vi "load_target.vi"() -> ()   [LabVIEW 2015]
uses:
  subvi/controls.llb/command.ctl
  <vilib>/Platform/TimedLoop/XDataNode/timing_clust.ctl
  <vilib>/Platform/TimedLoop/XDataNode/nitl_modes.ctl
  <vilib>/Platform/TimedLoop/XDataNode/wakeup.ctl
  subvi/controls.llb/RTFIFO operate.ctl
  subvi/Enum data queue_Ctrls.ctl
  <vilib>/addons/control/pid/pid.llb/PID (DBL).vi
  <vilib>/platform/TimedLoop/XDataNode/XDataNode.xnode
  subvi/event data queues.lvlib
  <vilib>/Platform/TimedLoop/XDataNode/XDNodeRunTimeDep.lvlib
  <vilib>/addons/control/pid/NI_PID_pid.lvlib
panel:
  out "T":dbl
  out "data":T1
  out "pat":T2
  out "Sin_MODE_RUN state 2":string
  out "Sin_MODE_RUN state":string
  out "doing":T3(ring)
  out "Boolean array":bool[](array[boolean])
  out "length 2":i32
  out "length":i32
  out "运行":string
  out "state":T3(ring)
  out "exit":bool=TRUE
  in  "variable":T5 {"command" items=["NO_Action", "start", "pause", "resum", "stop", "config"]}
  in  "error in":errorcluster
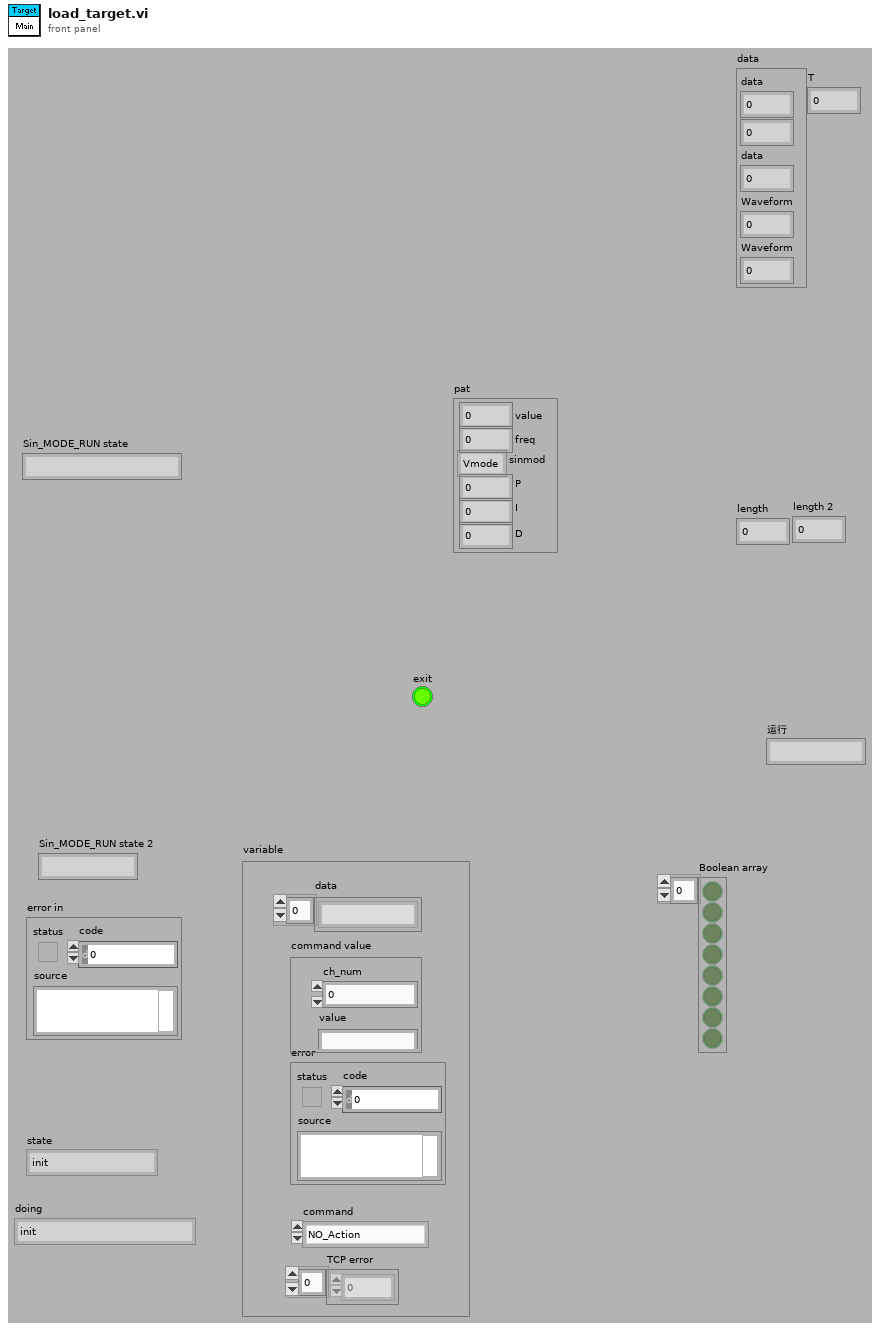
[diagram p1: front panel]
types:
  T1 = cluster{"data":dbl, dbl, "data":u8, "Waveform":dbl, "Waveform":dbl}
  T2 = cluster{"value":dbl, "freq":dbl, "sinmod":enum16{"Vmode", "Tmode", "PIDTmode"}, "P":dbl, "I":dbl, "\nD":dbl}
  T3 = enum16{"init", "wait", "start", "do", "stop", "exit"}
  T4 = typedef "command.ctl" = u16
  T5 = cluster{"error":errorcluster, "TCP error":i32[], "command":T4, "command value":cluster{"ch_num":dbl, "value":string}, "data":string[]}
  T6 = typedef "XDNodeRunTimeDep.lvlib/timing_clust.ctl" = cluster{"Expected End [f-1]":u64, "Actual End [f-1]":u64, "Finished Late? [f-1]":bool, "Expected End [i-1]":u64, "Actual End [i-1]":u64, "Finished Late? [i-1]":bool, "Expected Start [i]":u64, "Actual Start [i]":u64, "Expected Start [f]":u64, "Actual Start [f]":u64, "Source Name":string, "Structure Name":string, "Period":i64, "Deadline":i64, "Offset":i64, "Start":i64, "Priority":i32, "Timeout":i32, "Mode":T7, "Wakeup Reason":T8, "Error":errorcluster, "Source Type":string, "Secondary Source Type":string, "Global End Time":u64, "Global Start Time":u64, "Frame Duration":u64, "Iteration Duration":u64, "Assigned CPU":i32, "I/O Scan Engine Mode":u32}
  T7 = typedef "XDNodeRunTimeDep.lvlib/nitl_modes.ctl" = enum32{"No Change", "Process missed periods, maintain original phase", "Discard missed periods, maintain original phase", "Process missed periods, ignore original phase", "Discard missed periods, ignore original phase"}
  T8 = typedef "XDNodeRunTimeDep.lvlib/wakeup.ctl" = enum32{"Normal", "Aborted", "Asynchronous wakeup", "Timing source error", "Timed loop error", "Timeout"}
  T9 = enum16{"init", "config", "start", "write", "stop"}
  T10 = enum16{"init", "config", "start", "read", "stop"}
  T11 = enum16{"connect", "receive data", "send data", "data transfer", "close"}
  T12 = cluster{"data":dbl, dbl, "data":u8, dbl, "mean":dbl}
  T13 = cluster{"data":dbl, "seconds since 1Jan1904":timestamp}
  T14 = enum16{"connect", "receive data", "send data", "data transfer"}
  T15 = cluster{"value":dbl, "freq":dbl, "sinmod":enum16{"Vmode", "Tmode", "PIDTmode"}, "P":dbl, "I":dbl, "D":dbl}
  T16 = typedef "RTFIFO operate.ctl" = enum16{"Creat", "Write", "Read", "Delete"}
  T17 = typedef "event data queues.lvlib/Enum data queue_Ctrls.ctl" = enum16{"Noop", "Send Pro1", "Send data", "Get Pro1", "Get data", "Flush Pro1", "Flush data", "Destroy Pro1", "Destroy data"}
  T18 = cluster{"proportional gain (Kc)":dbl, "integral time (Ti, min)":dbl, "derivative time (Td, min)":dbl}
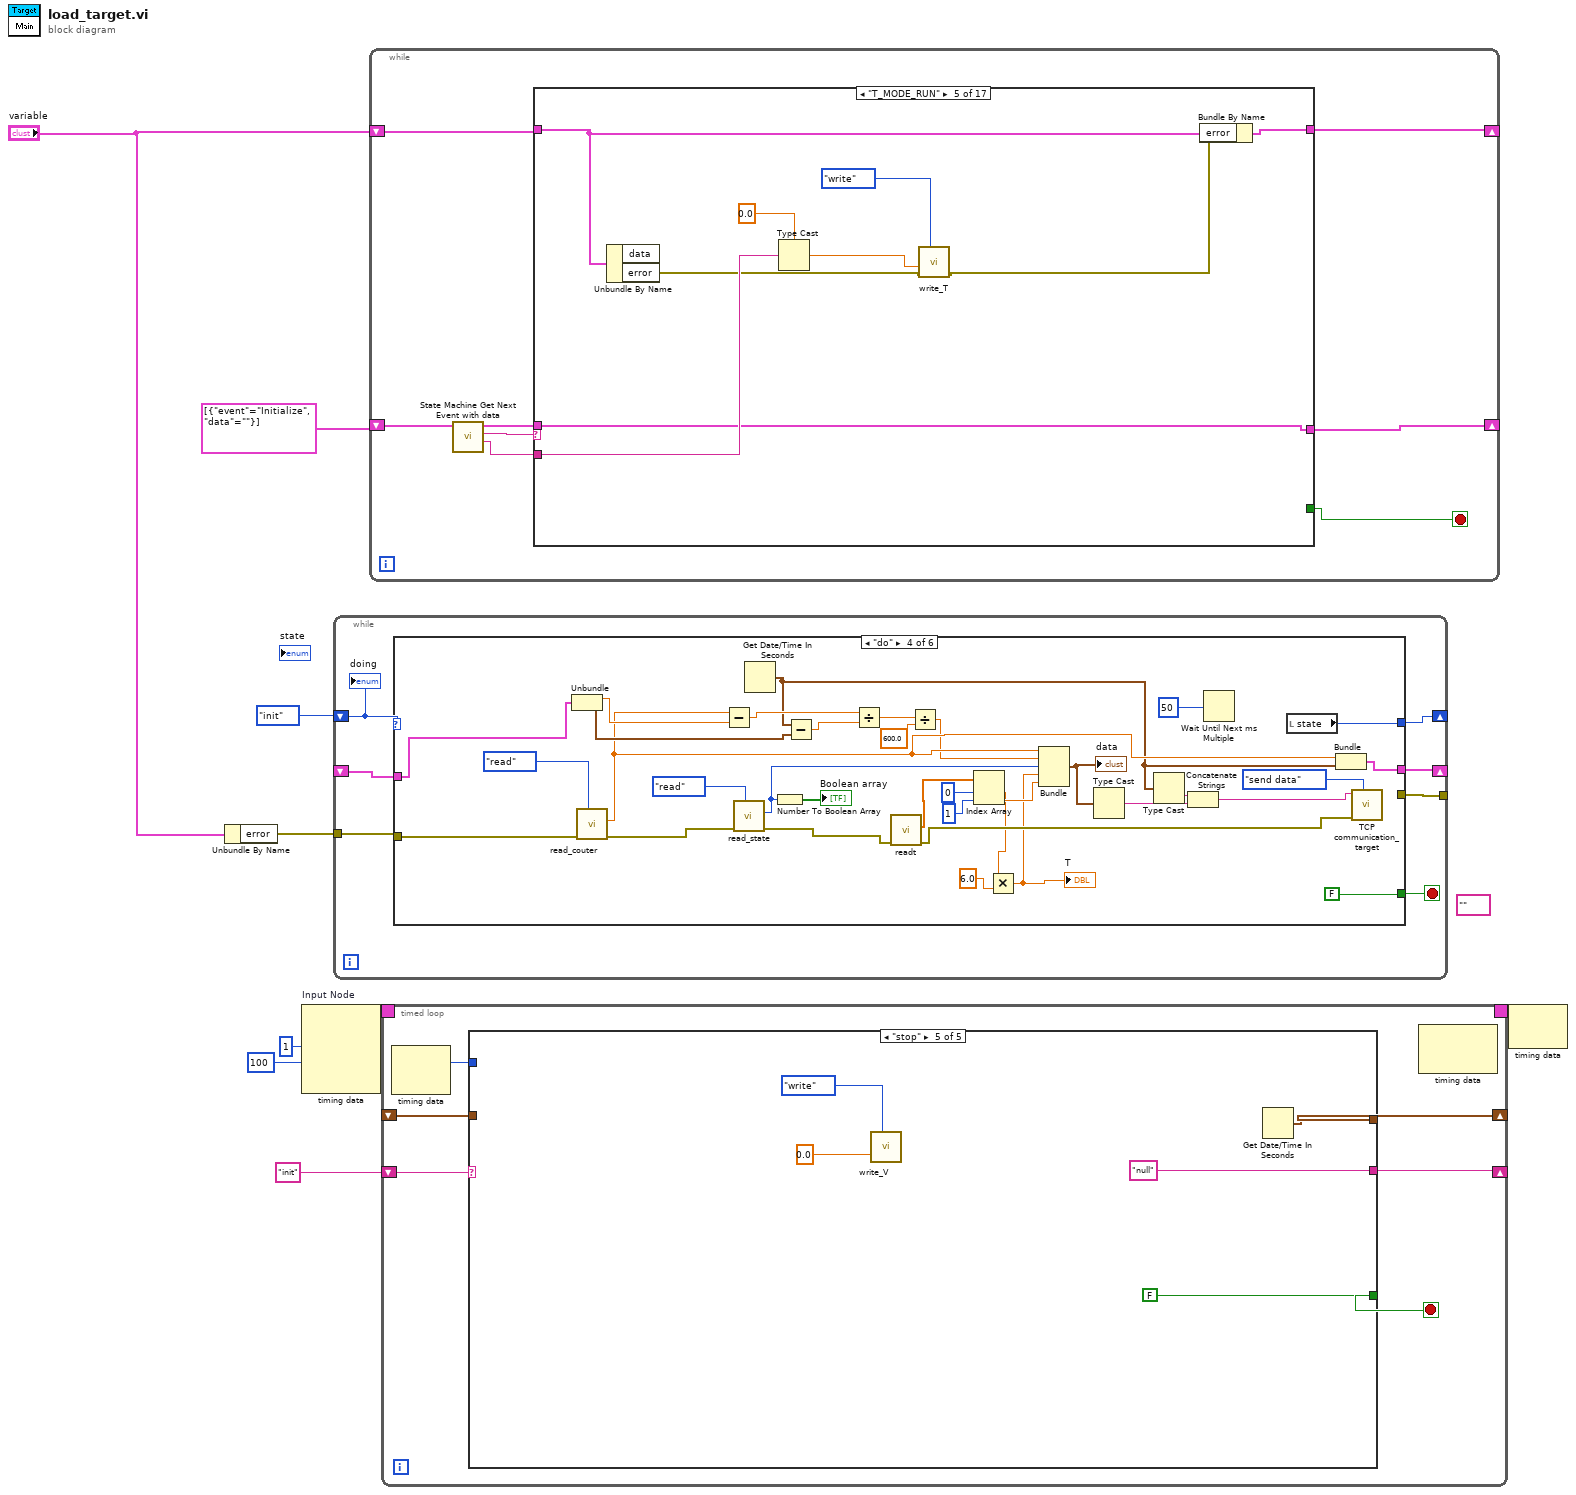
[diagram p0: block diagram]
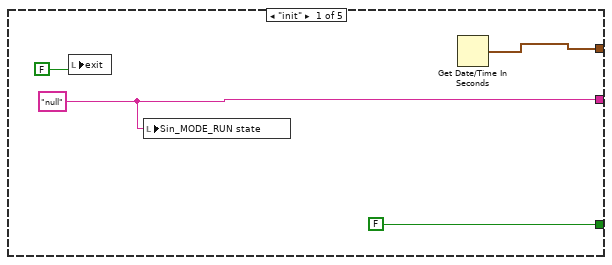
[diagram p2: hidden frame]
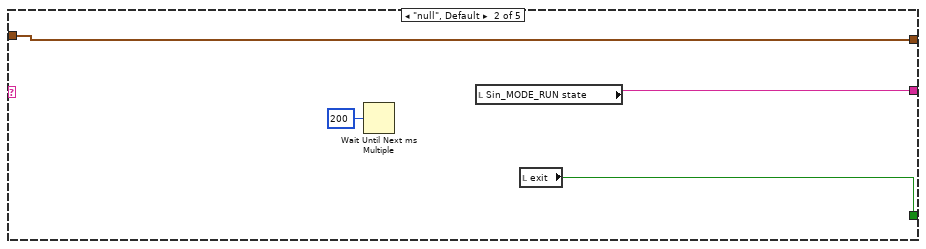
[diagram p3: hidden frame]
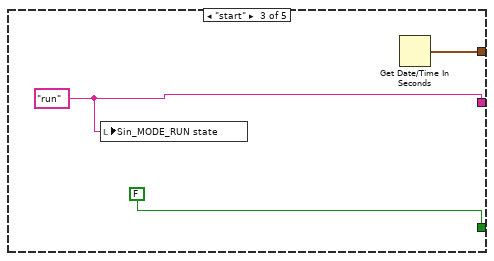
[diagram p4: hidden frame]
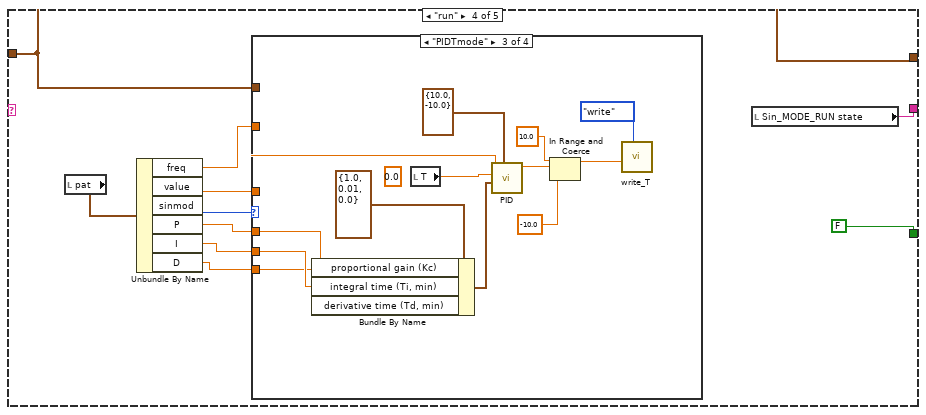
[diagram p5: hidden frame]
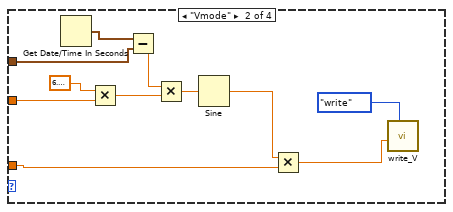
[diagram p7: hidden frame]
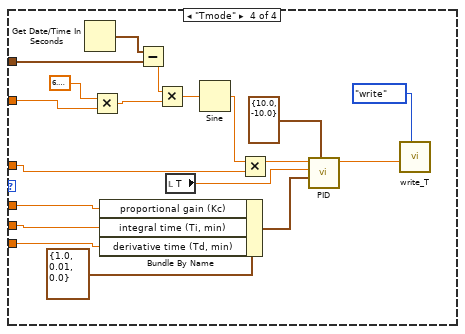
[diagram p8: hidden frame]
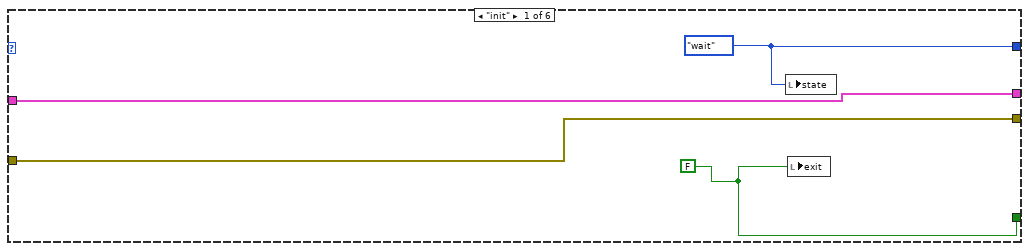
[diagram p9: hidden frame]
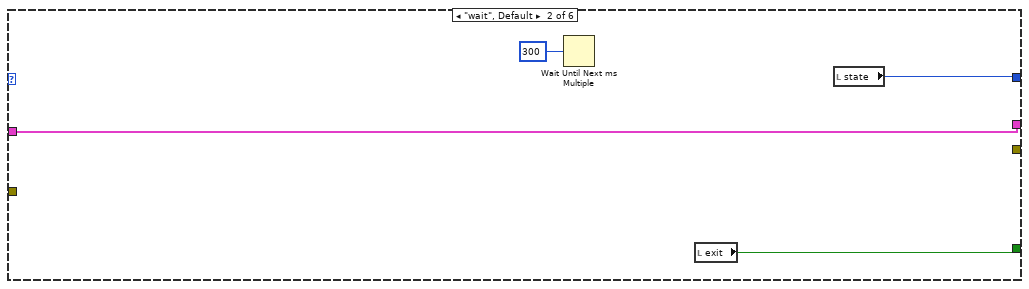
[diagram p10: hidden frame]
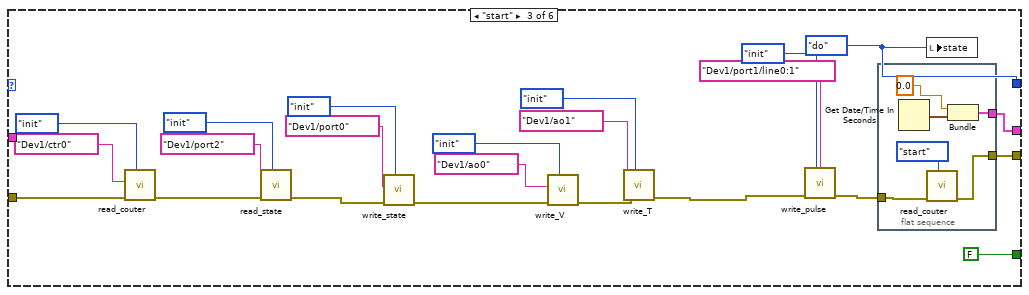
[diagram p11: hidden frame]
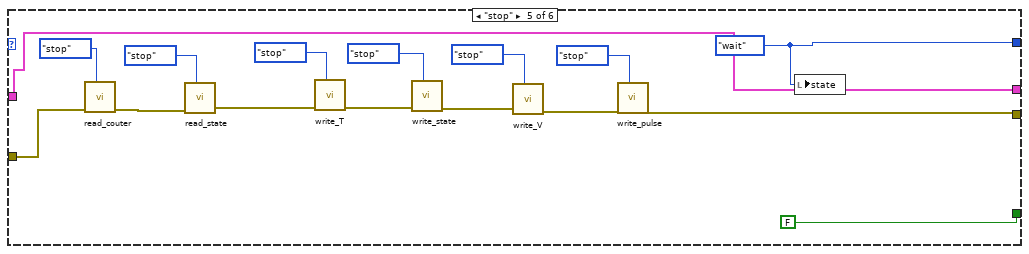
[diagram p12: hidden frame]
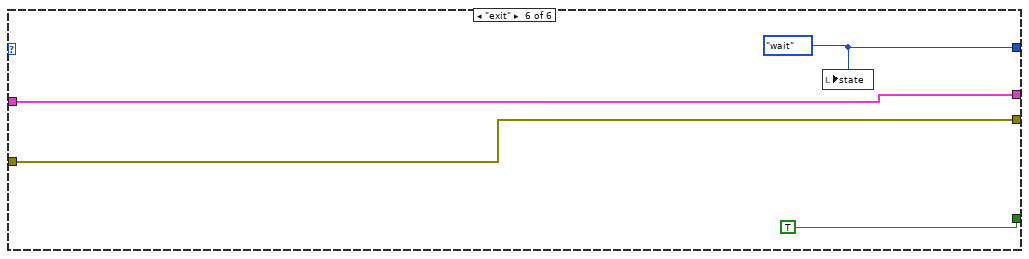
[diagram p13: hidden frame]
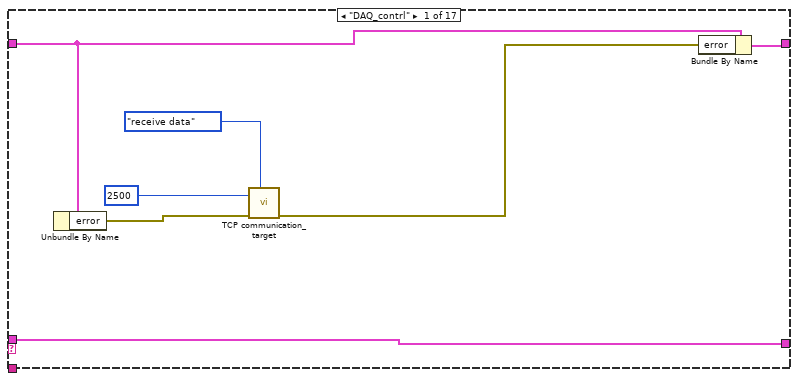
[diagram p14: hidden frame]
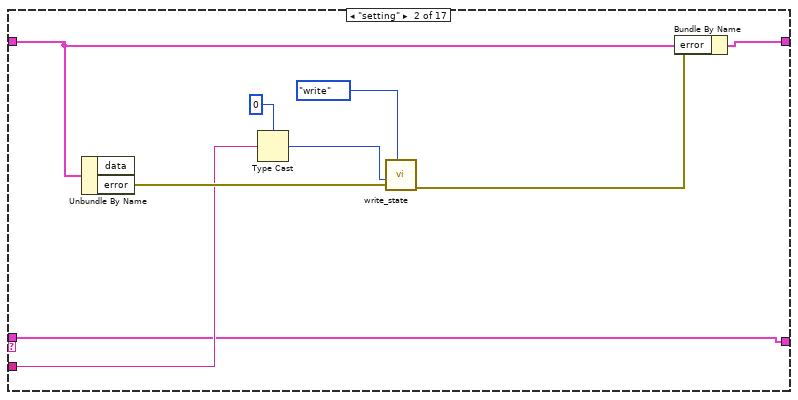
[diagram p15: hidden frame]
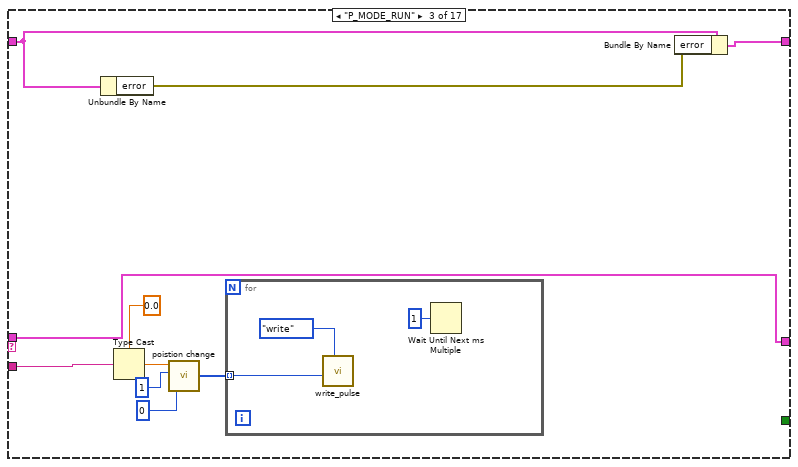
[diagram p16: hidden frame]
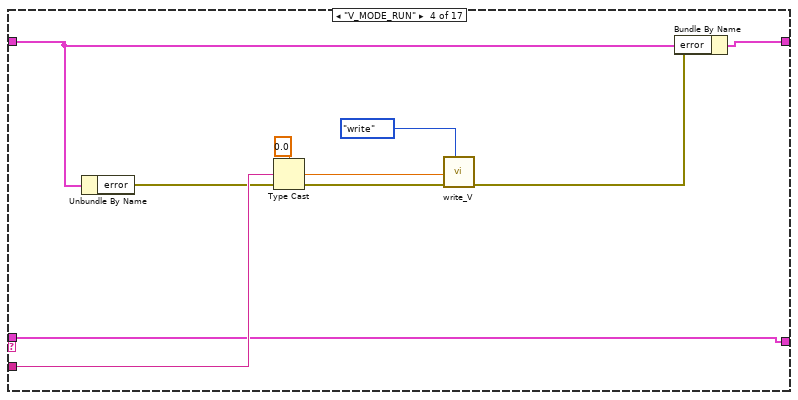
[diagram p17: hidden frame]
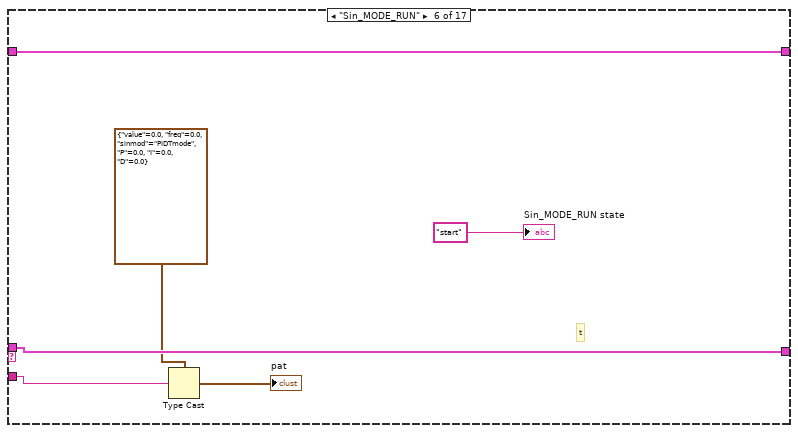
[diagram p18: hidden frame]
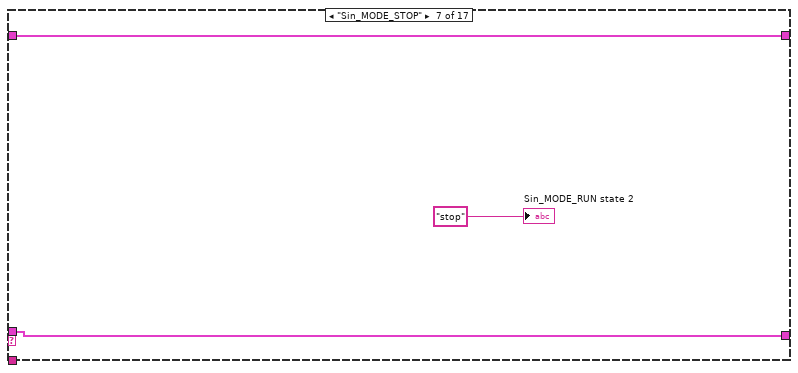
[diagram p19: hidden frame]
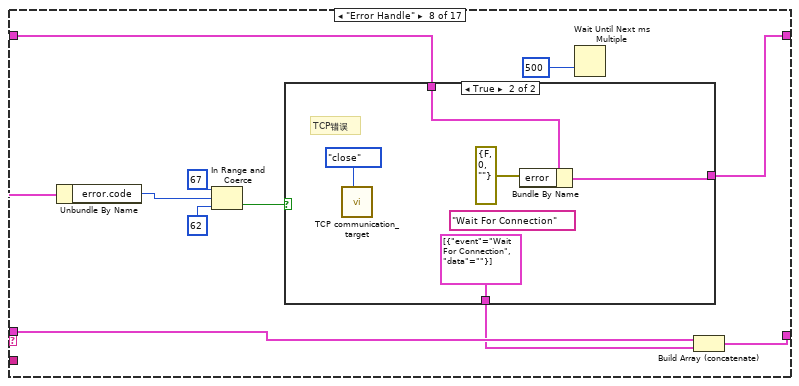
[diagram p20: hidden frame]
diagram:
  (unwired) tag "" ("physical channels")
  n1 = Unbundle By Name("variable") -> ("error"=w8:errorcluster)
  n2 = node-c288 "Input Node"(1 ("Priority"), i64 100 ("Period")) -> (w5:T6)  [unwired: 2 in]
  n3 = while {
    shift-right: [w14] -> _
    shift-left: T3."init" ("Enum") -> [w16]
    tunnel: w8 -> [w13]
    tunnel: [w12] -> _
    shift-right: [w11] -> _
    shift-left: _ -> [w10]
    stop <- w15 stop-if-true
    n4 = case shown="\"do\"" w16 {
      tunnel: [w20 w24 FALSE ("exit") FALSE ("exit") FALSE ("exit") TRUE ("exit")] -> w15
      tunnel: [w19 w23 w46 w86 w102 w106] -> w14
      tunnel: w13 -> [w18 _ w43 w85 w101 w105]
      tunnel: [w18 _ w35 _ w88 w105] -> w12
      tunnel: [w17 w21 w27 w69 w89 w104] -> w11
      tunnel: w10 -> [w17 w21 _ w73 w89 w104]
      frame "init" {
        w19 = T3."wait" ("Enum")
        w20 = FALSE
        n5 = local write "state"(w19) -> ()
        n6 = local write "exit"(w20) -> ()
      }
      frame "wait", Default {
        n7 = Wait Until Next ms Multiple(millisecond multiple=u32 300) -> ()  [unwired: 1 out]
        n8 = local read "exit"() -> (w24:bool)
        n9 = local read "state"() -> (w23:T3)
      }
      frame "start" {
        w46 = T3."do" ("Enum")
        n10 = call "read_couter.vi"("Enum"=T10."init", "error in"=w43, "counter"=tag "Dev1/ctr0") -> ("error out"=w36:errorcluster)  [unwired: 7 in, 1 out]
        n11 = call "read_state.vi"("Enum"=T10."init", "error in"=w36, "lines"=tag "Dev1/port2") -> ("error out"=w42:errorcluster)  [unwired: 7 in, 1 out]
        n12 = call "write_state.vi"("Enum"=T9."init", "error in"=w42, "lines"=tag "Dev1/port0") -> ("error out"=w40:errorcluster)  [unwired: 7 in]
        n13 = call "write_V.vi"("Enum"=T9."init", "error in"=w40, "physical channels"=tag "Dev1/ao0") -> ("error out"=w39:errorcluster)  [unwired: 8 in]
        n14 = call "write_T.vi"("Enum"=T9."init", "error in"=w39, "physical channels"=tag "Dev1/ao1") -> ("error out"=w25:errorcluster)  [unwired: 8 in]
        n15 = call "write_pulse.vi"("Enum"=T9."init", "error in"=w25, "lines"=tag "Dev1/port1/line0:1") -> ("error out"=w30:errorcluster)  [unwired: 7 in]
        n16 = flat-sequence {
          tunnel: [w53] -> w35
          tunnel: w30 -> [w51]
          tunnel: [w50] -> w27
          frame #0 {
            n17 = Get Date/Time In Seconds() -> (seconds since 1Jan1904=w49:timestamp)
            n18 = call "read_couter.vi"("Enum"=T10."start", "error in"=w51) -> ("error out"=w53:errorcluster)  [unwired: 8 in, 1 out]
            n19 = Bundle(0.0, "seconds since 1Jan1904"=w49) -> (w50:cluster{dbl, "seconds since 1Jan1904":timestamp})  [unwired: 1 in]
          }
        }
        n20 = local write "state"(w46) -> ()
      }
      frame "do" {
        n21 = Unbundle(w73) -> ("data"=w71:dbl, "seconds since 1Jan1904"=w72:timestamp)
        n22 = call "read_couter.vi"("Enum"=T10."read", "error in"=w85) -> ("error out"=w84:errorcluster, "data"=w68:dbl)  [unwired: 8 in]
        n23 = Subtract(x=w68, y=w71) -> (x-y=w70:dbl)
        n24 = call "read_state.vi"("Enum"=T10."read", "error in"=w84) -> ("error out"=w59:errorcluster, "data"=w81:u8)  [unwired: 8 in]
        n25 = Get Date/Time In Seconds() -> (seconds since 1Jan1904=w67:timestamp)
        n26 = Number To Boolean Array(number=w81) -> (Boolean array=→"Boolean array":bool[])
        n27 = Subtract(x=w67, y=w72) -> (x-y=w74:dbl)
        n28 = Divide(x=w70, y=w74) -> (x/y=w65:dbl)
        n29 = call "readt.vi"("error in"=w59) -> ("error out"=w58:errorcluster, "appended array"=w57:dbl[])  [unwired: 9 in]
        n30 = Divide(x=w65, y=600.0) -> (x/y=w66:dbl)
        n31 = Index Array(array=w57, index #1=0 ("index"), index #2=1 ("index")) -> (element #1=w56:dbl, element #2=w62:dbl)
        n32 = Multiply(x=w56, y=6.0 ("x")) -> (x*y=w54:dbl)
        "T" <- w54
        n33 = Bundle("data"=w68, w66, "data"=w81, w54, "mean"=w62) -> (w63:T12)  [unwired: 1 in]
        "data" <- w63
        n34 = Type Cast(x=w63) -> (*(type *) &x=w76:string)  [unwired: 1 in]
        n35 = Type Cast(x=w67) -> (*(type *) &x=w75:string)  [unwired: 1 in]
        n36 = Concatenate Strings(w75, w76) -> (w77:string)
        n37 = Wait Until Next ms Multiple(millisecond multiple=u32 50) -> ()  [unwired: 1 out]
        n38 = local read "state"() -> (w86:T3)
        n39 = Bundle("data"=w68, "seconds since 1Jan1904"=w67) -> (w69:T13)  [unwired: 1 in]
        n40 = call "TCP communication_target.vi"("TCP command"=T11."send data", "error in"=w58, "data in"=w77) -> ()  [unwired: 7 in, 2 out]
      }
      frame "stop" {
        w102 = T3."wait" ("Enum")
        n41 = call "read_couter.vi"("Enum"=T10."stop", "error in"=w101) -> ("error out"=w100:errorcluster)  [unwired: 8 in, 1 out]
        n42 = call "read_state.vi"("Enum"=T10."stop", "error in"=w100) -> ("error out"=w99:errorcluster)  [unwired: 8 in, 1 out]
        n43 = call "write_T.vi"("Enum"=T9."stop", "error in"=w99) -> ("error out"=w98:errorcluster)  [unwired: 9 in]
        n44 = call "write_state.vi"("Enum"=T9."stop", "error in"=w98) -> ("error out"=w93:errorcluster)  [unwired: 8 in]
        n45 = call "write_V.vi"("Enum"=T9."stop", "error in"=w93) -> ("error out"=w92:errorcluster)  [unwired: 9 in]
        n46 = call "write_pulse.vi"("Enum"=T9."stop", "error in"=w92) -> ("error out"=w88:errorcluster)  [unwired: 8 in]
        n47 = local write "state"(w102) -> ()
      }
      frame "exit" {
        w106 = T3."wait" ("Enum")
        n48 = local write "state"(w106) -> ()
      }
    }
    "doing" <- w16
  }
  n49 = while {
    shift-right: [w112] -> _
    shift-left: cluster{"event":string, "data":string}[] [{"event"="Initialize", "data"=""}] ("enent data queue in") -> [w109]
    shift-right: [w110] -> _
    shift-left: "variable" -> [w111]
    stop <- w114 stop-if-true
    n50 = call "State Machine Get Next Event with data.vi"("enent data queue in"=w109) -> ("data"=w108:string, "next event"=w115:string, "event queue out"=w113:cluster{"event":string, "data":string}[])  [unwired: 4 in]
    n51 = case shown="\"T_MODE_RUN\"" w115 {
      selector: w115 -> [_ _ _ _ _ _ _ _ _ _ w207 _ _ _ _ _ _]
      tunnel: [_ _ _ _ _ _ _ _ w194 _ _ _ _ _ _ _ _] -> w114
      tunnel: w113 -> [w120 w123 w132 w145 w154 w166 w169 w179 w193 w206 w209 w265 w273 w276 w282 _ w295]
      tunnel: [w120 w123 w132 w145 w154 w166 w169 w178 w193 w205 w208 w264 w272 w276 w281 w284 w294] -> w112
      tunnel: w111 -> [w118 w129 w141 w153 w162 w165 w170 w181 w192 w202 w212 w269 w271 w275 w279 w287 w293]
      tunnel: [w117 w128 w140 w152 w161 w165 w170 w180 w192 w201 w210 w269 w271 w275 w279 w287 w293] -> w110
      tunnel: w108 -> [_ w124 w138 w150 w159 w168 _ _ _ _ _ _ _ _ _ _ _]
      frame "DAQ_contrl" {
        n52 = Unbundle By Name(w118) -> ("error"=w119:errorcluster)
        n53 = call "TCP communication_target.vi"("TCP command"=T14."receive data", "error in"=w119, "timeout ms"=2500) -> ("error out"=w116:errorcluster)  [unwired: 7 in, 1 out]
        n54 = Bundle By Name(cluster=w118, "error"=w116) -> (w117:T5)
      }
      frame "setting" {
        n55 = Unbundle By Name(w129) -> ("error"=w130:errorcluster)  [unwired: 1 out]
        n56 = Type Cast(type=u8 0, x=w124) -> (*(type *) &x=w125:u8)
        n57 = call "write_state.vi"("Enum"=T9."write", "error in"=w130, "data"=w125) -> ("error out"=w127:errorcluster)  [unwired: 7 in]
        n58 = Bundle By Name(cluster=w129, "error"=w127) -> (w128:T5)
      }
      frame "P_MODE_RUN" {
        n59 = Unbundle By Name(w141) -> ("error"=w137:errorcluster)
        n60 = Type Cast(type=0.0, x=w138) -> (*(type *) &x=w136:dbl)
        n61 = call "poistion change.vi"("Value"=w136, "方向"=u32 1, "位置"=u32 0) -> ("Data"=w133:u8[])  [unwired: 6 in]
        n62 = for {
          tunnel: w133 -> [w143] mode=indexing
          n63 = call "write_pulse.vi"("Enum"=T9."write", "data"=w143) -> ()  [unwired: 8 in, 1 out]
          n64 = Wait Until Next ms Multiple(millisecond multiple=u32 1) -> ()  [unwired: 1 out]
        }
        n65 = Bundle By Name(cluster=w141, "error"=w137) -> (w140:T5)
      }
      frame "V_MODE_RUN" {
        n66 = Unbundle By Name(w153) -> ("error"=w149:errorcluster)
        n67 = Type Cast(type=0.0, x=w150) -> (*(type *) &x=w146:dbl)
        n68 = call "write_V.vi"("Enum"=T9."write", "error in"=w149, "Data"=w146) -> ("error out"=w148:errorcluster)  [unwired: 8 in]
        n69 = Bundle By Name(cluster=w153, "error"=w148) -> (w152:T5)
      }
      frame "T_MODE_RUN" {
        n70 = Unbundle By Name(w162) -> ("error"=w156:errorcluster)  [unwired: 1 out]
        n71 = Type Cast(type=0.0, x=w159) -> (*(type *) &x=w158:dbl)
        n72 = call "write_T.vi"("Enum"=T9."write", "error in"=w156, "Data"=w158) -> ("error out"=w155:errorcluster)  [unwired: 8 in]
        n73 = Bundle By Name(cluster=w162, "error"=w155) -> (w161:T5)
      }
      frame "Sin_MODE_RUN" {
        # "t"
        n74 = Type Cast(type=T15 {"value"=0.0, "freq"=0.0, "sinmod"=enum."PIDTmode", "P"=0.0, "I"=0.0, "D"=0.0}, x=w168) -> (*(type *) &x=→"pat":T15)
        "Sin_MODE_RUN state" <- "start"
      }
      frame "Sin_MODE_STOP" {
        "Sin_MODE_RUN state 2" <- "stop"
      }
      frame "Error Handle" {
        n75 = Unbundle By Name(w181) -> ("error.code"=w177:i32)
        n76 = In Range and Coerce(upper limit=67, x=w177, lower limit=62) -> (In Range?=w174:bool)  [unwired: 1 out]
        n77 = case shown="True" w174 {
          tunnel: w181 -> [w184 w188]
          tunnel: [w182 w187] -> w180
          tunnel: [_ cluster{"event":string, "data":string}[] [{"event"="Wait For Connection", "data"=""}] ("array")] -> w173
          frame False {
            n78 = Bundle By Name(cluster=w184, "error"=errorcluster {"status"=FALSE, "code"=0, "source"=""}) -> (w182:T5)
          }
          frame True {
            (unwired) "Wait For Connection"
            # "TCP错误"
            n79 = call "TCP communication_target.vi"("TCP command"=T11."close") -> ()  [unwired: 9 in, 2 out]
            n80 = Bundle By Name(cluster=w188, "error"=errorcluster {"status"=FALSE, "code"=0, "source"=""}) -> (w187:T5)
          }
        }
        n81 = Wait Until Next ms Multiple(millisecond multiple=u32 500) -> ()  [unwired: 1 out]
        n82 = Build Array (concatenate)(w179, w173) -> (w178:cluster{"event":string, "data":string}[])
      }
      frame "Exit" {
        w194 = TRUE
        n83 = Wait Until Next ms Multiple(millisecond multiple=u32 500) -> ()  [unwired: 1 out]
        n84 = local write "state"(T3."wait" ("Enum")) -> ()
        "exit" <- w194
      }
      frame "Initialize" {
        w199 = 66 items=["No Error", "Argument Error", "Memory Full", "Out of Zone", "End of File", "File Already Open", "Generic File IO Error", "File Not Found", "File Permission Error", "Disk Full", "Duplicate Path", "Too Many Files Open", "Not Enabled", "Resource File Not Found", "Cannot Add Resource", "Resource Not Found", "Image Not Found", "Image Memory Error", "Pen Does Not Exist", "Config Bad Type", "Config Token Not Found", "Config Parse Error", "Config Memory Error", "Bad External Code Format", "Bad External Code Offset", "External Code Not Present", "Null Window", "Destroy Window Mixup", "Null Menu", "Print Aborted", "Bad Print Record", "Print Driver Error", "Windows Error During Print", "Memory Error During Print", "Print Dialog Error", "Generic Print Error", "Invalid Device Refnum", "Device Not Found", "Device Parameter Error", "Device Unit Error", "Can't Open Device", "Device Call Aborted", "Generic Error", "Cancelled By User", "Object ID Too Low", "Object ID Too High", "Object Not In Heap", "Unknown Heap", "Bad DefProc ID", "DefProc Not In Table", "Message Out Of Range", "Null Method", "Unknown Message", "Manager Call Not Supported", "Bad address", "Connection In progress", "Connection timed out", "Connection is already in progress", "Network attribute not supported", "Network error", "Address in use", "System out of memory", "Connection aborted", "Connection refused", "Connection is not connected", "Connection is already connected", "Connection closed", "Initialize error (interapplication manager)", "Bad occurrence", "Wait on unbound occurrence handler", "Occurrence queue overflow", "Bad path", "Semaphore not signaled", "Unrecognized type (interapplication manager)"] ("1st Error to Convert")
        w198 = 56 items=["No Error", "Argument Error", "Memory Full", "Out of Zone", "End of File", "File Already Open", "Generic File IO Error", "File Not Found", "File Permission Error", "Disk Full", "Duplicate Path", "Too Many Files Open", "Not Enabled", "Resource File Not Found", "Cannot Add Resource", "Resource Not Found", "Image Not Found", "Image Memory Error", "Pen Does Not Exist", "Config Bad Type", "Config Token Not Found", "Config Parse Error", "Config Memory Error", "Bad External Code Format", "Bad External Code Offset", "External Code Not Present", "Null Window", "Destroy Window Mixup", "Null Menu", "Print Aborted", "Bad Print Record", "Print Driver Error", "Windows Error During Print", "Memory Error During Print", "Print Dialog Error", "Generic Print Error", "Invalid Device Refnum", "Device Not Found", "Device Parameter Error", "Device Unit Error", "Can't Open Device", "Device Call Aborted", "Generic Error", "Cancelled By User", "Object ID Too Low", "Object ID Too High", "Object Not In Heap", "Unknown Heap", "Bad DefProc ID", "DefProc Not In Table", "Message Out Of Range", "Null Method", "Unknown Message", "Manager Call Not Supported", "Bad address", "Connection In progress", "Connection timed out", "Connection is already in progress", "Network attribute not supported", "Network error", "Address in use", "System out of memory", "Connection aborted", "Connection refused", "Connection is not connected", "Connection is already connected", "Connection closed", "Initialize error (interapplication manager)", "Bad occurrence", "Wait on unbound occurrence handler", "Occurrence queue overflow", "Bad path", "Semaphore not signaled", "Unrecognized type (interapplication manager)"] ("1st Error to Convert")
        w200 = 64 items=["No Error", "Argument Error", "Memory Full", "Out of Zone", "End of File", "File Already Open", "Generic File IO Error", "File Not Found", "File Permission Error", "Disk Full", "Duplicate Path", "Too Many Files Open", "Not Enabled", "Resource File Not Found", "Cannot Add Resource", "Resource Not Found", "Image Not Found", "Image Memory Error", "Pen Does Not Exist", "Config Bad Type", "Config Token Not Found", "Config Parse Error", "Config Memory Error", "Bad External Code Format", "Bad External Code Offset", "External Code Not Present", "Null Window", "Destroy Window Mixup", "Null Menu", "Print Aborted", "Bad Print Record", "Print Driver Error", "Windows Error During Print", "Memory Error During Print", "Print Dialog Error", "Generic Print Error", "Invalid Device Refnum", "Device Not Found", "Device Parameter Error", "Device Unit Error", "Can't Open Device", "Device Call Aborted", "Generic Error", "Cancelled By User", "Object ID Too Low", "Object ID Too High", "Object Not In Heap", "Unknown Heap", "Bad DefProc ID", "DefProc Not In Table", "Message Out Of Range", "Null Method", "Unknown Message", "Manager Call Not Supported", "Bad address", "Connection In progress", "Connection timed out", "Connection is already in progress", "Network attribute not supported", "Network error", "Address in use", "System out of memory", "Connection aborted", "Connection refused", "Connection is not connected", "Connection is already connected", "Connection closed", "Initialize error (interapplication manager)", "Bad occurrence", "Wait on unbound occurrence handler", "Occurrence queue overflow", "Bad path", "Semaphore not signaled", "Unrecognized type (interapplication manager)"] ("1st Error to Convert")
        (unwired) "Wait For Connection"
        n85 = Build Array (concatenate)(w206, cluster{"event":string, "data":string} {"event"="Wait For Connection", "data"=""} ("enent data queue in")) -> (w205:cluster{"event":string, "data":string}[])
        n86 = Build Array(w200, w199, w198) -> (w197:i32[])
        n87 = call "RTFIFO Model.vi"("size"=4000, "operate"=RTFIFO_operate."Creat") -> ("error out"=w196:errorcluster)  [unwired: 8 in, 1 out]
        n88 = Bundle By Name(cluster=w202, "TCP error"=w197, "error"=w196) -> (w201:T5)
      }
      frame "Default", Default {
        n89 = Unbundle By Name(w212) -> ("error.status"=w211:bool)
        n90 = case shown="True" w211 {
          tunnel: [w221 w256] -> w210
          tunnel: w212 -> [w220 w256]
          tunnel: w209 -> [w219 w255]
          tunnel: [w218 w254] -> w208
          frame False {
            n91 = call "TCP communication_target.vi"("TCP command"=T14."receive data", "timeout ms"=300) -> ("error out"=w216:errorcluster, "Data out"=w217:string[])  [unwired: 8 in]
            n92 = Unbundle By Name(w216) -> ("code"=w215:i32)
            n93 = Equal?(x=w215, y=56) -> (x = y?=w213:bool)
            n94 = case shown="False" w213 {
              tunnel: [w235 w251] -> w221
              tunnel: w220 -> [w234 w251]
              tunnel: w219 -> [w230 w250]
              tunnel: [w229 w250] -> w218
              tunnel: w217 -> [w226 _]
              tunnel: w216 -> [w227 _]
              frame False {
                n95 = call "convert tcp data (host command).vi"("error in"=w227, "TCP Data"=w226) -> ("error out"=w233:errorcluster, "command"=w228:T4)  [unwired: 8 in]
                n96 = Index Array "Index Array"(array=w226, index=1) -> (element=w224:string)
                n97 = call "case according to command.vi"("error in"=w233, "command"=w228) -> ("error out"=w232:errorcluster, "case"=w231:string)  [unwired: 8 in]
                n98 = case shown="0, Default" w228 {
                  tunnel: w230 -> [w241 w248]
                  tunnel: [w240 w246] -> w229
                  tunnel: w231 -> [w237 w245]
                  tunnel: w224 -> [w236 w242]
                  frame 0, Default {
                    n99 = Bundle By Name(cluster=cluster{"event":string, "data":string} {"event"="", "data"=""} ("new element/subarray"), "event"=w237, "data"=w236) -> (w239:cluster{"event":string, "data":string})
                    n100 = Build Array (concatenate)(w241, w239) -> (w240:cluster{"event":string, "data":string}[])
                  }
                  frame 13 {
                    n101 = Bundle By Name(cluster=cluster{"event":string, "data":string} {"event"="", "data"=""} ("new element/subarray"), "event"=w245, "data"=w242) -> (w243:cluster{"event":string, "data":string})
                    n102 = Insert Into Array "Insert Into Array"(array=w248, index=0, new element=w243) -> (w246:cluster{"event":string, "data":string}[])
                  }
                }
                n103 = Bundle By Name(cluster=w234, "data"=w226, "command"=w228, "error"=w232) -> (w235:T5)
              }
              frame True {
                n104 = Wait Until Next ms Multiple(millisecond multiple=u32 500) -> ()  [unwired: 1 out]
              }
            }
          }
          frame True {
            # "DAQ_read"
            n105 = Wait Until Next ms Multiple(millisecond multiple=u32 500) -> ()  [unwired: 1 out]
            n106 = Build Array (concatenate)(w255, cluster{"event":string, "data":string} {"event"="Error Handle", "data"=""} ("enent data queue in")) -> (w254:cluster{"event":string, "data":string}[])
          }
        }
        "运行" <- w207
      }
      frame "Wait For Connection" {
        n107 = call "TCP communication_target.vi"("TCP command"=T14."connect", "error in"="error in", "remote port"=u16 6342, "timeout ms"=500) -> ("error out"=w266:errorcluster)  [unwired: 6 in, 1 out]
        n108 = Select(t="Wait For Connection", s=w266, f="Default") -> (s? t:f=w259:string)
        n109 = Bundle By Name(cluster=cluster{"event":string, "data":string} {"event"="", "data"=""} ("new element/subarray"), "event"=w259) -> (w261:cluster{"event":string, "data":string})
        n110 = Build Array (concatenate)(w265, w261) -> (w264:cluster{"event":string, "data":string}[])
      }
      frame "DAQ_init" {
        n111 = Build Array (concatenate)(w273, cluster{"event":string, "data":string} {"event"="DAQ_config", "data"=""} ("new element/subarray")) -> (w272:cluster{"event":string, "data":string}[])
      }
      frame "DAQ_config" {
        n112 = Wait Until Next ms Multiple(millisecond multiple=u32 500) -> ()  [unwired: 1 out]
      }
      frame "DAQ_start" {
        n113 = local write "state"(T3."start" ("Enum")) -> ()
        n114 = Build Array (concatenate)(w282, cluster{"event":string, "data":string} {"event"="DAQ_read", "data"=""} ("new element/subarray")) -> (w281:cluster{"event":string, "data":string}[])
        n115 = Wait Until Next ms Multiple(millisecond multiple=u32 500) -> ()  [unwired: 1 out]
      }
      frame "DAQ_stop" {
        n116 = local write "state"(T3."stop" ("Enum")) -> ()
        n117 = Wait Until Next ms Multiple(millisecond multiple=u32 500) -> ()  [unwired: 1 out]
        n118 = Build Array(cluster{"event":string, "data":string} {"event"="Default", "data"=""} ("new element/subarray")) -> (w284:cluster{"event":string, "data":string}[])
      }
      frame "DAQ_read" {
        n119 = call "Event data  Queues Manager.vi"("Mode"=Enum_data_queue_Ctrls."Get data") -> ("data"=w289:cluster{"time":timestamp, "data":string}, "timed out?"=w288:bool, "error out"=w290:errorcluster)  [unwired: 11 in, 1 out]
        n120 = case shown="True" w288 {
          tunnel: w290 -> [w303 _]
          tunnel: w289 -> [w302 _]
          frame False {
            n121 = Unbundle By Name(w302) -> ("time"=w301:timestamp, "data"=w296:string)
            n122 = Type Cast(x=w301) -> (*(type *) &x=w297:string)  [unwired: 1 in]
            n123 = String Length(string=w297) -> (length=→"length":i32)
            n124 = String Length(string=w296) -> (length=→"length 2":i32)
            n125 = Concatenate Strings(w297, w296) -> (w300:string)
            n126 = call "TCP communication_target.vi"("TCP command"=T11."send data", "error in"=w303, "data in"=w300) -> ()  [unwired: 7 in, 2 out]
          }
          frame True {
          }
        }
        n127 = Build Array (concatenate)(w295, cluster{"event":string, "data":string}[] [{"event"="No Action", "data"=""}, {"event"="DAQ_read", "data"=""}]) -> (w294:cluster{"event":string, "data":string}[])
      }
    }
  }
  n128 = timed-loop {
    timing: w5 -> [_]
    timing-out: [_] -> w4
    shift-right: [w308] -> _
    shift-left: "init" -> [w310]
    shift-right: [w307] -> _
    shift-left: _ -> [w306]
    stop <- w309 stop-if-true
    n129 = node-c288() -> (w305:i64)  [unwired: 1 in, 1 out]
    n130 = case shown="\"stop\"" w310 {
      tunnel: [FALSE ("exit") w318 FALSE ("exit") FALSE ("exit") FALSE ("exit")] -> w309
      tunnel: [w313 w317 w320 w330 "null" ("Sin_MODE_RUN state")] -> w308
      tunnel: [w311 w315 w319 w322 w375] -> w307
      tunnel: w306 -> [_ w315 _ w322 _]
      tunnel: w305 -> [_ _ _ _ _]
      frame "init" {
        w313 = "null"
        n131 = local write "exit"(FALSE) -> ()
        n132 = local write "Sin_MODE_RUN state"(w313) -> ()
        n133 = Get Date/Time In Seconds() -> (seconds since 1Jan1904=w311:timestamp)
      }
      frame "null", Default {
        n134 = Wait Until Next ms Multiple(millisecond multiple=u32 200) -> ()  [unwired: 1 out]
        n135 = local read "Sin_MODE_RUN state"() -> (w317:string)
        n136 = local read "exit"() -> (w318:bool)
      }
      frame "start" {
        w320 = "run"
        n137 = local write "Sin_MODE_RUN state"(w320) -> ()
        n138 = Get Date/Time In Seconds() -> (seconds since 1Jan1904=w319:timestamp)
      }
      frame "run" {
        n139 = local read "pat"() -> (w329:T2)
        n140 = Unbundle By Name(w329) -> ("freq"=w326:dbl, "value"=w327:dbl, "sinmod"=w328:enum16{"Vmode", "Tmode", "PIDTmode"}, "P"=w325:dbl, "I"=w324:dbl, "D"=w323:dbl)
        n141 = case shown="\"PIDTmode\"" w328 {
          tunnel: w327 -> [_ w337 w354 w370]
          tunnel: w326 -> [_ w336 _ w369]
          tunnel: w325 -> [_ _ w346 w363]
          tunnel: w324 -> [_ _ w345 w362]
          tunnel: w323 -> [_ _ w344 w361]
          tunnel: w322 -> [_ w333 _ w357]
          frame Default {
          }
          frame "Vmode" {
            n142 = Get Date/Time In Seconds() -> (seconds since 1Jan1904=w334:timestamp)
            n143 = Multiply(x=6.283185307179586, y=w336) -> (x*y=w340:dbl)
            n144 = Subtract(x=w334, y=w333) -> (x-y=w332:dbl)
            n145 = Multiply(x=w332, y=w340) -> (x*y=w339:dbl)
            n146 = Sine(x=w339) -> (sin(x)=w338:dbl)
            n147 = Multiply(x=w338, y=w337) -> (x*y=w335:dbl)
            n148 = call "write_V.vi"("Enum"=T9."write", "Data"=w335) -> ()  [unwired: 9 in, 1 out]
          }
          frame "PIDTmode" {
            (unwired) 0.0 ("T")
            n149 = Bundle By Name(cluster=T18 {"proportional gain (Kc)"=1.0, "integral time (Ti, min)"=0.01, "derivative time (Td, min)"=0.0} ("PID gains"), "proportional gain (Kc)"=w346, "integral time (Ti, min)"=w345, "derivative time (Td, min)"=w344) -> (w343:T18)
            n150 = local read "T"() -> (w349:dbl)
            n151 = call-poly <vilib>:"PID.vi"("output range"=cluster{"output high":dbl, "output low":dbl} {"output high"=10.0, "output low"=-10.0}, "PID gains"=w343, "process variable"=w349, "setpoint"=w354) -> ("output"=w352:dbl)  [unwired: 6 in, 1 out]
            n152 = In Range and Coerce(upper limit=10.0, x=w352, lower limit=-10.0) -> (coerced(x)=w348:dbl)  [unwired: 1 out]
            n153 = call "write_T.vi"("Enum"=T9."write", "Data"=w348) -> ()  [unwired: 9 in, 1 out]
          }
          frame "Tmode" {
            n154 = Get Date/Time In Seconds() -> (seconds since 1Jan1904=w358:timestamp)
            n155 = Multiply(x=6.283185307179586, y=w369) -> (x*y=w373:dbl)
            n156 = Bundle By Name(cluster=T18 {"proportional gain (Kc)"=1.0, "integral time (Ti, min)"=0.01, "derivative time (Td, min)"=0.0} ("PID gains"), "proportional gain (Kc)"=w363, "integral time (Ti, min)"=w362, "derivative time (Td, min)"=w361) -> (w364:T18)
            n157 = Subtract(x=w358, y=w357) -> (x-y=w356:dbl)
            n158 = Multiply(x=w356, y=w373) -> (x*y=w372:dbl)
            n159 = local read "T"() -> (w359:dbl)
            n160 = Sine(x=w372) -> (sin(x)=w371:dbl)
            n161 = Multiply(x=w371, y=w370) -> (x*y=w367:dbl)
            n162 = call-poly <vilib>:"PID.vi"("output range"=cluster{"output high":dbl, "output low":dbl} {"output high"=10.0, "output low"=-10.0}, "PID gains"=w364, "process variable"=w359, "setpoint"=w367) -> ("output"=w360:dbl)  [unwired: 6 in, 1 out]
            n163 = call "write_T.vi"("Enum"=T9."write", "Data"=w360) -> ()  [unwired: 9 in, 1 out]
          }
        }
        n164 = local read "Sin_MODE_RUN state"() -> (w330:string)
      }
      frame "stop" {
        n165 = call "write_V.vi"("Enum"=T9."write", "Data"=0.0) -> ()  [unwired: 9 in, 1 out]
        n166 = Get Date/Time In Seconds() -> (seconds since 1Jan1904=w375:timestamp)
      }
    }
    n167 = node-c288() -> ()  [unwired: 2 in, 1 out]
  }
  n168 = node-c288(w4) -> ()  [unwired: 1 out]
